vi "ELVIS III v1.0 Close AI Block.vi"(8 "error in (no error)":errorcluster, 10 "AI (N Samples) Channels List":T1, 11 "myRIO AI (N Samples) Ref In":T3) -> (0 "error out":errorcluster)   [LabVIEW 2021]
uses:
  <vilib>/myRIO/Common/Instrument Driver Framework/Utilities/typedefs/myRIO v1.0 Reference.ctl
  <vilib>/myRIO/Common/Instrument Driver Framework/Utilities/typedefs/Generic FPGA Reference.ctl
  <vilib>/myRIO/Common/Instrument Driver Framework/myRIO v1.0/AI Block/typedefs/AI Block Channels List.ctl
  <vilib>/myRIO/Common/Instrument Driver Framework/myRIO v1.0/AI Block/typedefs/AI Block Channels Enum.ctl
  <vilib>/myRIO/Common/Instrument Driver Framework/ELVIS III v1.0/AI Block/vis/ELVIS III v1.0 Build MUX Configuration AI Block.vi
  <vilib>/myRIO/Common/Instrument Driver Framework/ELVIS III v1.0/Resource Manager/vis/ELVIS III v1.0 Unreserve Channel List.vi
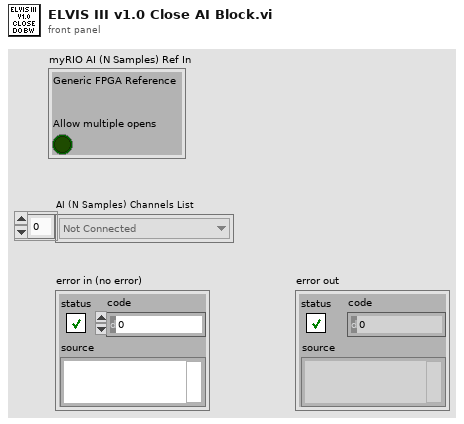
[diagram p1: front panel]
types:
  T1 = typedef "AI Block Channels List.ctl" = T2[]
  T2 = typedef "AI Block Channels Enum.ctl" = enum16{"Not Connected", "A/AI0 (N Samples)", "A/AI1 (N Samples)", "A/AI2 (N Samples)", "A/AI3 (N Samples)", "A/AI4 (N Samples)", "A/AI5 (N Samples)", "A/AI6 (N Samples)", "A/AI7 (N Samples)", "A/AI0 (DIFF N Samples)", "A/AI1 (DIFF N Samples)", "A/AI2 (DIFF N Samples)", "A/AI3 (DIFF N Samples)", "B/AI0 (N Samples)", "B/AI1 (N Samples)", "B/AI2 (N Samples)", "B/AI3 (N Samples)", "B/AI4 (N Samples)", "B/AI5 (N Samples)", "B/AI6 (N Samples)", "B/AI7 (N Samples)", "B/AI0 (DIFF N Samples)", "B/AI1 (DIFF N Samples)", "B/AI2 (DIFF N Samples)", "B/AI3 (DIFF N Samples)"}
  T3 = typedef "myRIO v1.0 Reference.ctl" = cluster{"Generic FPGA Reference":T4, "Allow multiple opens":bool}
  T4 = typedef "Generic FPGA Reference.ctl" = refnum<k20>
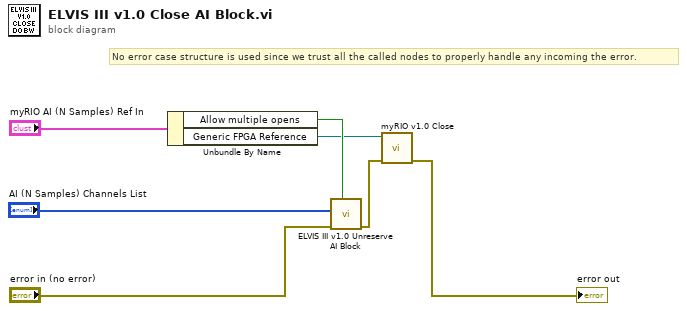
[diagram p0: block diagram]
diagram:
  # "No error case structure is used since we trust all the called nodes to properly handle any incoming the error."
  n1 = Unbundle By Name("myRIO AI (N Samples) Ref In") -> ("Allow multiple opens"=w3:bool, "Generic FPGA Reference"=w1:T4)
  n2 = call <vilib>:"ELVIS III v1.0 Unreserve AI Block.vi"("Allow multiple opens?"=w3, "error in (no error)"="error in (no error)", "AI (N Samples) Channels List"="AI (N Samples) Channels List") -> ("error out"=w6:errorcluster)  [unwired: 8 in]
  n3 = call <vilib>:"myRIO v1.0 Close.vi"("error in (no error)"=w6, "myRIO FPGA Ref In"=w1) -> ("error out"=→"error out":errorcluster)  [unwired: 9 in]
